vi "HeartRateMonitor.vi"() -> ()   [LabVIEW 2010]
panel:
  in  "Frequency":dbl(slide) scale=1.0..10.0
  in  "Threshold Voltage":dbl=3.183
  out "Waveform Chart":dynamicdata(graph)
  out "Amplitude Value":dbl
  out "Final Pulse Count":dbl
  out "Temp Pulse Count":dbl
  out "FLAG":dbl
  out "PulseDetected":bool
  out "BPM":dbl
  out "Timeout":bool
  out "Elapsed Time":dbl
  out "Out of range Alert":bool
  in  "stop":bool
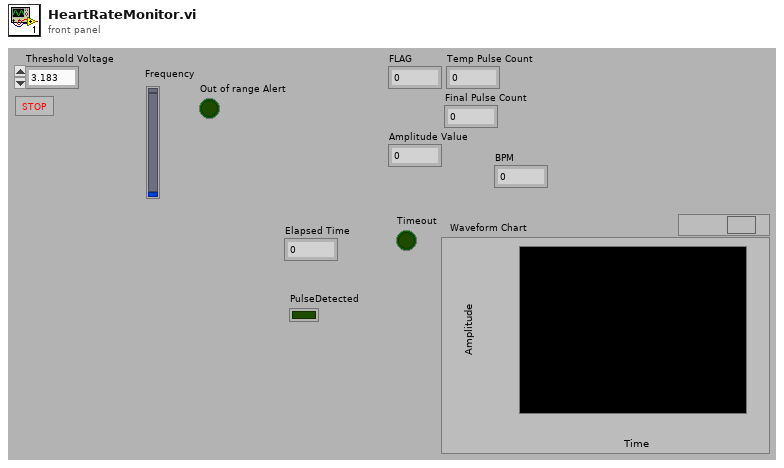
[diagram p1: front panel]
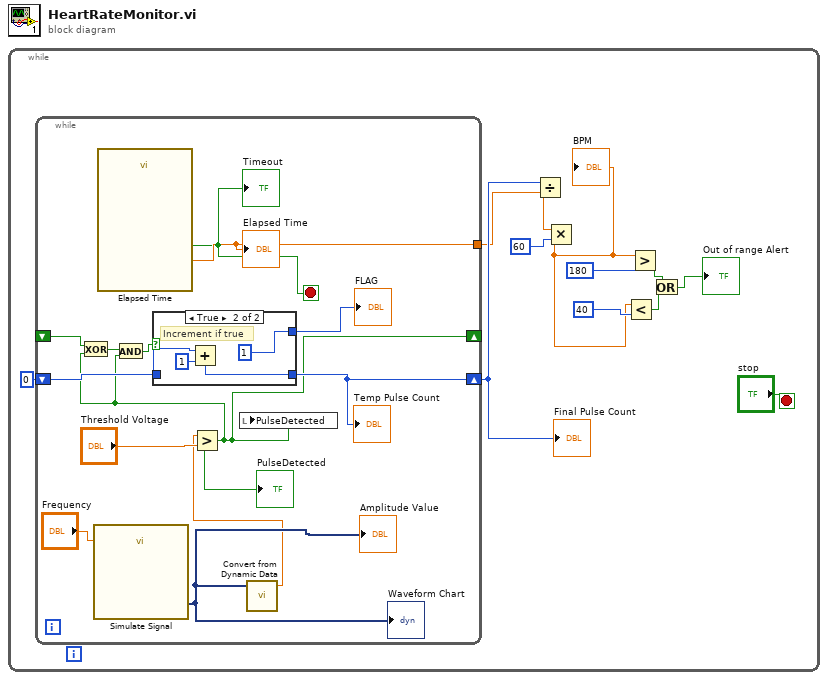
[diagram p0: block diagram]
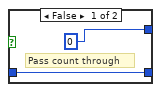
[diagram p2: hidden frame]
diagram:
  n1 = while {
    stop <- "stop" stop-if-true
    n2 = while {
      tunnel: [w25] -> w1
      shift-right: [w16] -> _
      shift-left: _ -> [w22]
      shift-right: [w19] -> w2
      shift-left: 0 -> [w20]
      stop <- w24 stop-if-true
      n3 = call "Simulate Signal"("Frequency"="Frequency") -> ("Sine"=w14:dynamicdata)  [unwired: 13 in, 1 out]
      "Amplitude Value" <- w14
      "Waveform Chart" <- w14
      n4 = call "Elapsed Time"() -> ("Elapsed Time (s)"=w25:dbl, "Time has Elapsed"=w24:bool)  [unwired: 12 in, 6 out]
      "Elapsed Time" <- w25
      "Timeout" <- w24
      n5 = call "Convert from Dynamic Data"("Dynamic Data Type"=w14) -> ("Scalar"=w13:dbl)  [unwired: 3 in]
      n6 = Greater?(x=w13, y="Threshold Voltage") -> (0:w16:bool)
      "PulseDetected" <- w16
      n7 = Exclusive Or(1:w16, 2:w22) -> (0:w17:bool)
      n8 = And(x=w17, y=w16) -> (x .and. y?=w18:bool)
      n9 = case shown="True" w18 {
        tunnel: [0 1] -> w21
        tunnel: [w26 w29] -> w19
        tunnel: w20 -> [w26 w28]
        frame False {
          # "Pass count through"
        }
        frame True {
          # "Increment if true"
          n10 = Add(x=w28, y=1) -> (x+y=w29:i32)
        }
      }
      "FLAG" <- w21
      "Temp Pulse Count" <- w19
      n11 = local write "PulseDetected"(w16) -> ()
    }
    "Final Pulse Count" <- w2
    n12 = Divide(x=w2, y=w1) -> (x/y=w5:dbl)
    n13 = Multiply(x=w5, y=60) -> (x*y=w4:dbl)
    "BPM" <- w4
    n14 = Less?(x=w4, y=40) -> (x < y?=w7:bool)
    n15 = Greater?(x=w4, y=180) -> (0:w11:bool)
    n16 = Or(x=w11, y=w7) -> (x .or. y?=→"Out of range Alert":bool)
  }
